vi "Call FP Cleanup.vi"(0 "VI":refnum<vi>, 11 "error in (no error)":errorcluster) -> (15 "error out":errorcluster)   [LabVIEW 2021, in "Converter Reusables.lvlib"]
uses:
  Converter Reusables.lvlib
  Dummy.vi
  Path Functions/Path Functions.lvlib
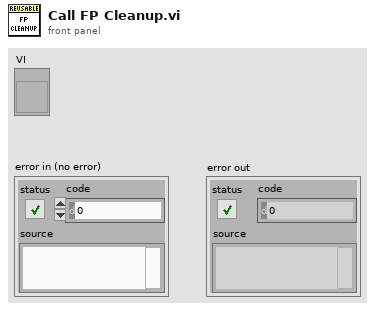
[diagram p1: front panel]
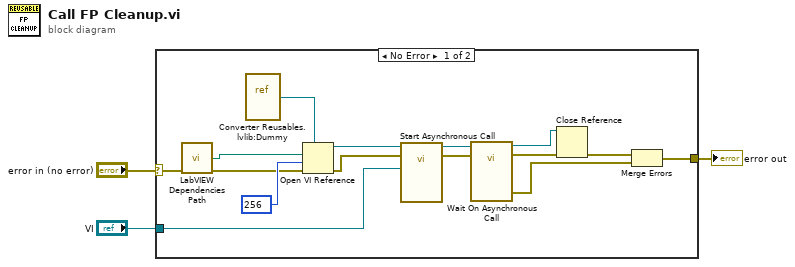
[diagram p0: block diagram]
diagram:
  n1 = case shown="No Error" "error in (no error)" {
    selector: "error in (no error)" -> [w4 w19]
    tunnel: "VI" -> [w14 _]
    tunnel: [w10 w19] -> w2
    frame No Error {
      n2 = call "LabVIEW Dependencies Path.vi"("error in (no error)"=w4) -> ("Arrange FP Path"=w6:path, "error out"=w5:errorcluster)  [unwired: 11 in, 2 out]
      n3 = vi-ref "Converter Reusables.lvlib:Dummy.vi"() -> (w17:refnum<vi>)
      n4 = Open VI Reference(type specifier VI Refnum (for type only)=w17, vi path=w6, options=256, error in (no error)=w5) -> (vi reference=w16:refnum<vi>, error out=w15:errorcluster)  [unwired: 2 in]
      n5 = call-by-ref "Start Asynchronous Call"(reference=w16, error in=w15, "VI"=w14) -> (reference out=w13:refnum<vi>, error out=w12:errorcluster)  [unwired: 14 in, 1 out]
      n6 = call-by-ref "Wait On Asynchronous Call"(reference=w13, error in=w12) -> (reference out=w7:refnum<vi>, error out=w9:errorcluster, 15:"error out"=w11:errorcluster)  [unwired: 15 in]
      n7 = Close Reference(reference=w7, error in (no error)=w9) -> (error out=w8:errorcluster)
      n8 = Merge Errors(w8, w11) -> (w10:errorcluster)
    }
    frame Error {
    }
  }
  "error out" <- w2
